vi "meas_timing.vi"() -> (1 "meas cycle time":u32)   [LabVIEW 2011]
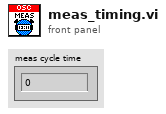
[diagram p1: front panel]
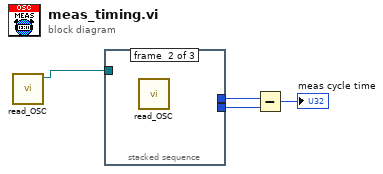
[diagram p0: block diagram]
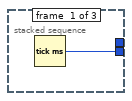
[diagram p2: hidden frame]
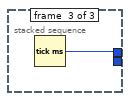
[diagram p3: hidden frame]
diagram:
  n1 = call "read_OSC.vi"() -> ("VISA resource name out"=w4:refnum<visa-resource-name>)  [unwired: 8 in, 3 out]
  n2 = stacked-sequence {
    tunnel: w4 -> [_ _ _]
    tunnel: [w5 _ _] -> w2
    tunnel: [_ _ w6] -> w3
    frame #0 {
      n3 = Tick Count (ms)() -> (millisecond timer value=w5:u32)
    }
    frame #1 {
      n4 = call "read_OSC.vi"() -> ()  [unwired: 8 in, 4 out]
    }
    frame #2 {
      n5 = Tick Count (ms)() -> (millisecond timer value=w6:u32)
    }
  }
  n6 = Subtract(x=w3, y=w2) -> (x-y=→"meas cycle time":u32)
